vi "Insight_IDN.vi"(8 "error in (no error)":errorcluster, 11 "telnet connection":T1) -> (0 "error out":errorcluster, 2 "*IDN?":string, 3 "telnet  connection out":T1)   [LabVIEW 2014]
doc: "Insight Photonic Solutions\n\nThis VI sends a *IDN? command to the laser and returns the laser identification information.\n\nver 1.0 - original release"
uses:
  Telnet Session.ctl
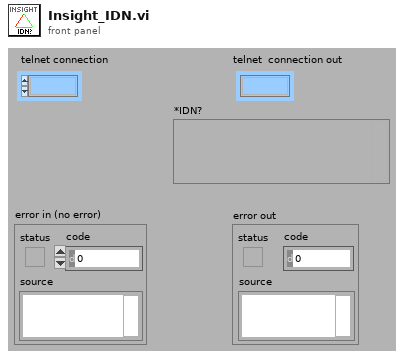
[diagram p1: front panel]
types:
  T1 = typedef "Telnet Session.ctl" = refnum<k1>
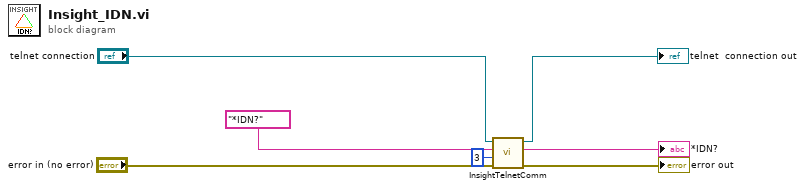
[diagram p0: block diagram]
diagram:
  n1 = call "InsightTelnetComm.vi"("error in"="error in (no error)", "Timeout, sec"=u32 3, "write buffer (\"\")"="*IDN?" ("String"), "telnet connection"="telnet connection") -> ("error out"=→"error out":errorcluster, "response data"=→"*IDN?":string, "telnet  connection out"=→"telnet  connection out":T1)  [unwired: 3 in]
